vi "Validate Coil Mapping.vi"(8 "error in (no error)":errorcluster, 10 "Mapping":u16) -> (0 "error out":errorcluster, 1 "Status Message":string, 3 "Valid?":bool)   [LabVIEW 2015]
uses:
  Modbus Master System Explorer.lvlib
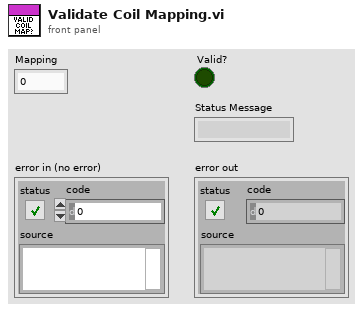
[diagram p1: front panel]
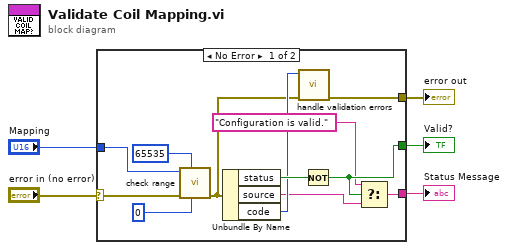
[diagram p0: block diagram]
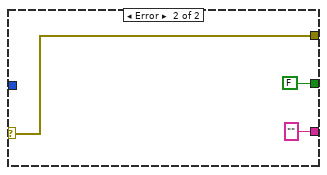
[diagram p2: hidden frame]
diagram:
  n1 = case shown="No Error" "error in (no error)" {
    selector: "error in (no error)" -> [w9 w20]
    tunnel: "Mapping" -> [w6 _]
    tunnel: [w15 w20] -> w3
    tunnel: [w14 FALSE] -> w2
    tunnel: [w11 "" ("source")] -> w1
    frame No Error {
      n2 = call "check range.vi"("lower limit"=0, "upper limit"=65535, "error in (no error)"=w9, "Mapping"=w6) -> ("error out"=w10:errorcluster)  [unwired: 7 in]
      n3 = Unbundle By Name(w10) -> ("status"=w17:bool, "source"=w12:string, "code"=w16:i32)
      n4 = call "handle validation errors.vi"("error in (no error)"=w10, "code"=w16) -> ("error out"=w15:errorcluster)  [unwired: 9 in]
      n5 = Not(x=w17) -> (.not. x?=w14:bool)
      n6 = Select(t="Configuration is valid." ("source"), s=w14, f=w12) -> (s? t:f=w11:string)
    }
    frame Error {
    }
  }
  "error out" <- w3
  "Valid?" <- w2
  "Status Message" <- w1
